vi "Wait For Compile.vi"(11 "FPGAtarget in":refnum<class "FPGATarget.lvclass">) -> (0 "compiled":bool, 3 "FPGAtarget out":refnum<class "FPGATarget.lvclass">)   [LabVIEW 2020, in "NI_TargetHelper.lvlib" / "FPGATarget.lvclass"]
uses:
  <vilib>/TargetSupport/NI_TargetHelper/FPGATarget/FPGATarget.lvclass
  <vilib>/TargetSupport/NI_TargetHelper/FPGATarget/FPGATarget.lvclass/FPGATarget.ctl
  <vilib>/TargetSupport/NI_TargetHelper/NI_TargetHelper.lvlib
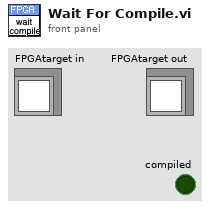
[diagram p1: front panel]
types:
  T1 = typedef "NI_TargetHelper.lvlib/Instance VIref.ctl" = refnum<vi>
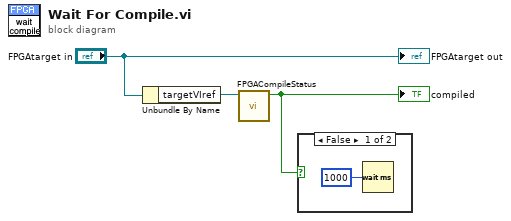
[diagram p0: block diagram]
diagram:
  n1 = Unbundle By Name("FPGAtarget in") -> ("targetVIref"=w2:T1)
  n2 = call <vilib>:"FPGACompileStatus.vi"("targetVIref"=w2) -> ("compile done"=w1:bool)  [unwired: 8 in, 2 out]
  "compiled" <- w1
  n3 = case shown="False" w1 {
    frame False {
      n4 = Wait (ms)(milliseconds to wait=u32 1000) -> ()  [unwired: 1 out]
    }
    frame True {
    }
  }
  "FPGAtarget out" <- "FPGAtarget in"
